vi "BcAppInfo.vi"(8 "error in (no error)":errorcluster, 10 "AppOutputData":T1, 11 "ModuleID":i32) -> (0 "error out":errorcluster)   [LabVIEW 2014, in "AppModule.lvlib"]
uses:
  AppModule.lvlib
  PublicAPI/Arguments/Requests/BC_AppInfo.ctl
  Framework/BusController/Admin/Registry/BCReg.lvclass
  clEventType.ctl
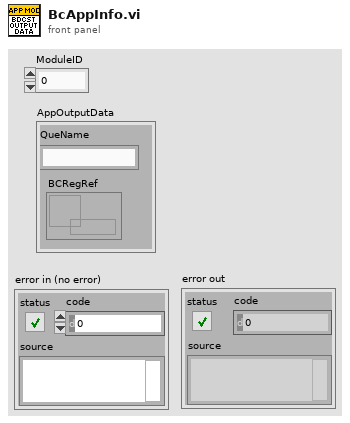
[diagram p1: front panel]
types:
  T1 = typedef "AppModule.lvlib/BC_AppInfo.ctl" = cluster{"QueName":string, "BCRegRef":refnum<data-value>}
  T2 = typedef "AppModule.lvlib/clEventType.ctl" = cluster{"ModuleID":i32, "Data":variant}
  T3 = typedef "AppModule.lvlib/clBroadcastEvents.ctl" = cluster{"DidInit":refnum<user-event>, "StatusUpdate":refnum<user-event>, "ErrorReport":refnum<user-event>, "DidStop":refnum<user-event>, "PathToINI":refnum<user-event>, "InputData":refnum<user-event>, "OutputData":refnum<user-event>, "BcAppInfo":refnum<user-event>, "ConfigData":refnum<user-event>}
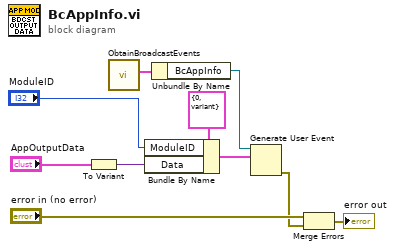
[diagram p0: block diagram]
diagram:
  n1 = To Variant(anything="AppOutputData") -> (Variant=w1:variant)
  n2 = call "ObtainBroadcastEvents.vi"() -> ("AppModuleBroadcast"=w8:T3)  [unwired: 10 in, 1 out]
  n3 = Bundle By Name(cluster=T2 {"ModuleID"=0, "Data"=variant} ("clEventType"), "ModuleID"="ModuleID", "Data"=w1) -> (w7:T2)
  n4 = Unbundle By Name(w8) -> ("BcAppInfo"=w6:refnum<user-event>)
  n5 = Generate User Event(user event=w6, event data cluster=w7) -> (error out=w3:errorcluster)  [unwired: 2 in, 1 out]
  n6 = Merge Errors("error in (no error)", w3) -> (→"error out":errorcluster)
